vi "Batch-Import-User-Channels Group.vi"(8 "error in (no error)":errorcluster, 11 "Node Ptr":T1 format="%.0x") -> (0 "error out":errorcluster)   [LabVIEW 2015, in "Batch-Import-User-Channels Custom Device.lvlib"]
uses:
  Batch-Import-User-Channels Custom Device.lvlib
  <vilib>/NI Veristand/Custom Device API/Custom Device Item Ref.ctl
  <vilib>/NI Veristand/Custom Device API/Custom Device Channel.ctl
  <vilib>/NI Veristand/Custom Device API/Custom Device Channel Type.ctl
  <vilib>/NI Veristand/Custom Device API/Custom Device API.lvlib
panel:
  in  "Add Channel Folder":bool
  in  "Add Channel":bool
  in  "Header":cluster{"Section Name":string}={"Section Name"="Item Settings"}
  in  "Description":string
  in  "Name":string
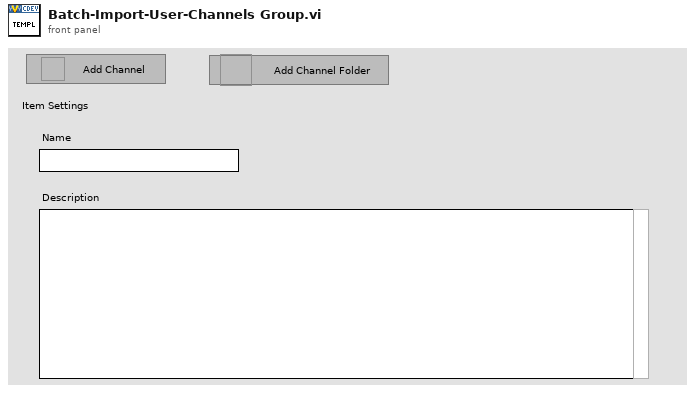
[diagram p1: front panel]
types:
  T1 = typedef "Custom Device API.lvlib/Custom Device Item Ref.ctl" = u64
  T2 = typedef "Custom Device API.lvlib/Custom Device Item Info.ctl" = cluster{"Name":string, "Is Channel":bool, "GUID":string, "Is Waveform":bool}
  T3 = typedef "Custom Device API.lvlib/Custom Device Channel.ctl" = cluster{"Type":T4, "Units":string, "Default Value":dbl, "Faultable":bool, "Scalable":bool}
  T4 = typedef "Custom Device API.lvlib/Custom Device Channel Type.ctl" = enum16{"Input", "Output"}
  T5 = typedef "Custom Device API.lvlib/Custom Device Commands.ctl" = enum16{"Default", "Item renamed", "Shutdown", "Dynamic button pressed"}
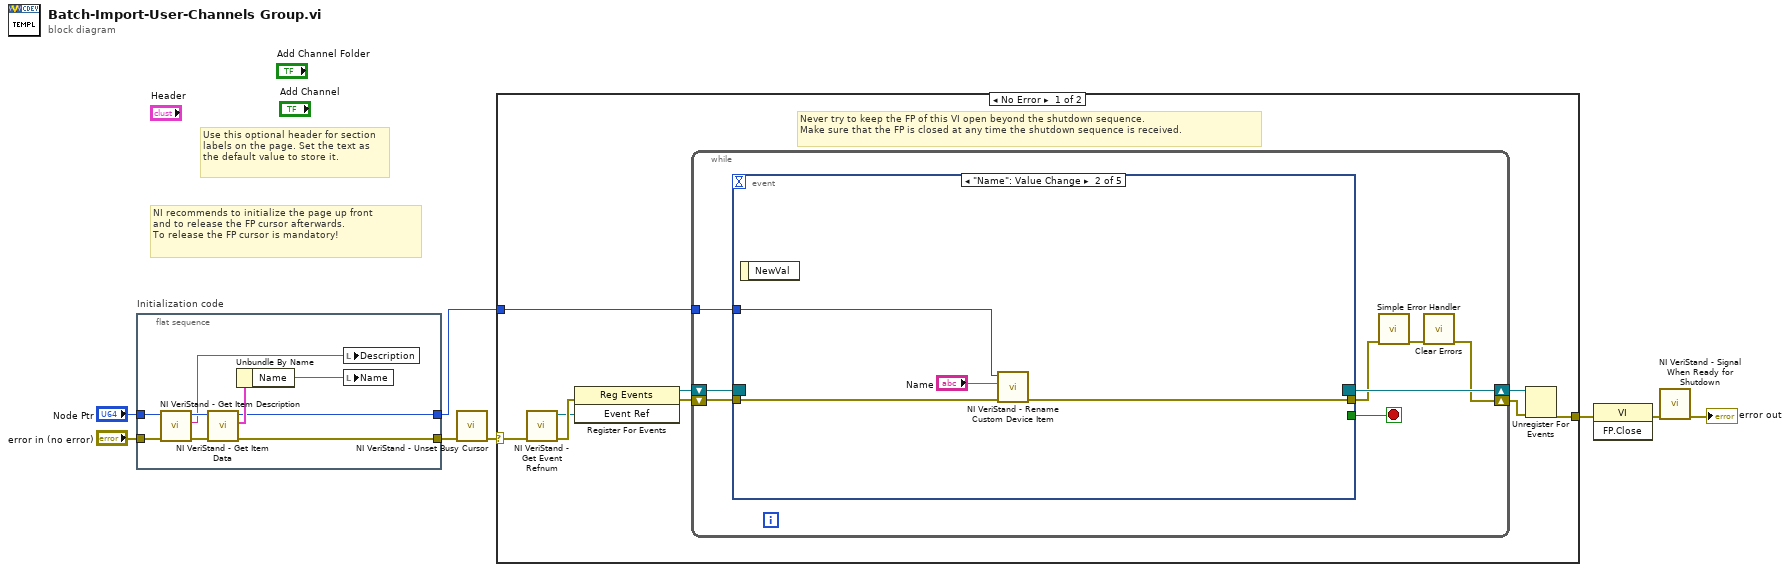
[diagram p0: block diagram]
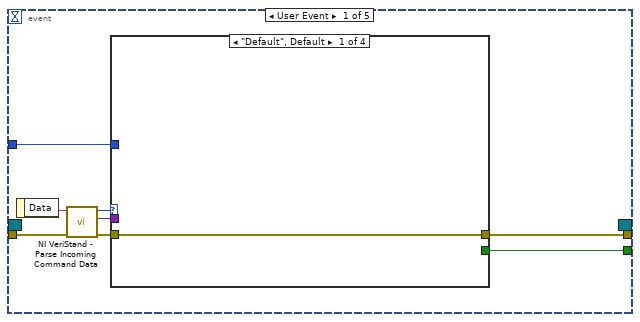
[diagram p2: hidden frame]
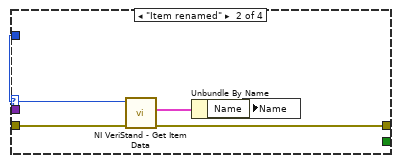
[diagram p3: hidden frame]
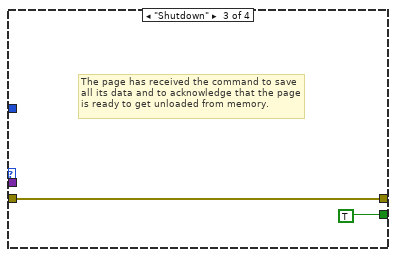
[diagram p4: hidden frame]
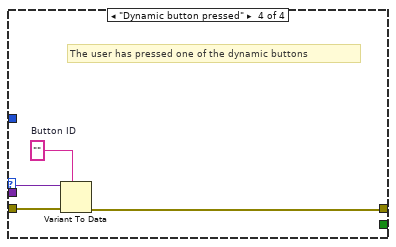
[diagram p5: hidden frame]
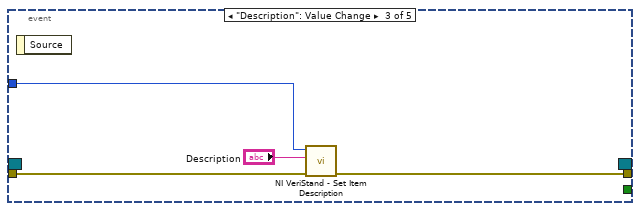
[diagram p6: hidden frame]
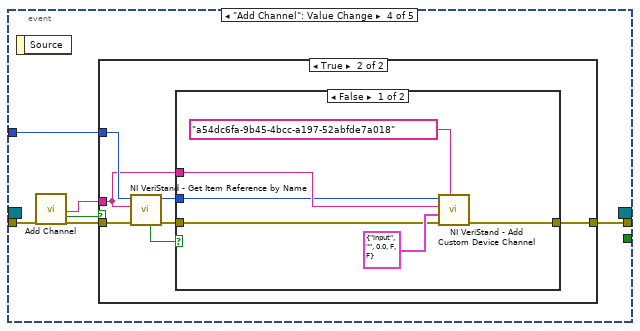
[diagram p7: hidden frame]
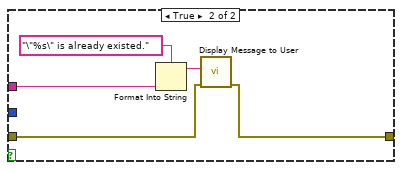
[diagram p9: hidden frame]
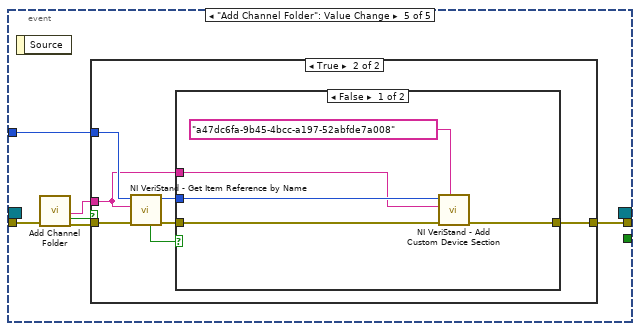
[diagram p10: hidden frame]
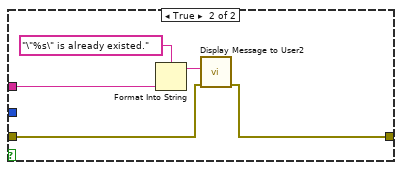
[diagram p12: hidden frame]
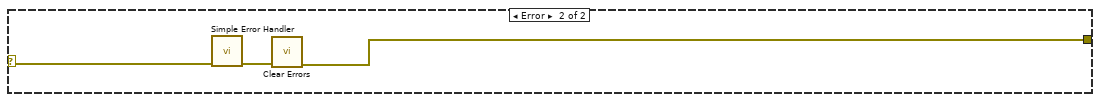
[diagram p13: hidden frame]
diagram:
  # "Use this optional header for section labels on the page. Set the text as the default value to store it."
  # "NI recommends to initialize the page up front\nand to release the FP cursor afterwards.\nTo release the FP cursor is mandatory!"
  n1 = flat-sequence "Initialization code" {
    tunnel: "error in (no error)" -> [w16]
    tunnel: "Node Ptr" -> [w15]
    tunnel: [w9] -> w2
    tunnel: [w10] -> w1
    frame #0 {
      n2 = call <vilib>:"NI VeriStand - Get Item Description.vi"("error in (no error)"=w16, "Item Ref in"=w15) -> ("error out"=w13:errorcluster, "Description"=w14:string, "Item Ref out"=w17:T1)  [unwired: 7 out]
      n3 = call <vilib>:"NI VeriStand - Get Item Data.vi"("error in (no error)"=w13, "Item Ref in"=w17) -> ("error out"=w9:errorcluster, "Item Info"=w12:T2, "Item Ref out"=w10:T1)  [unwired: 7 out]
      n4 = Unbundle By Name(w12) -> ("Name"=w11:string)
      n5 = local write "Description"(w14) -> ()
      n6 = local write "Name"(w11) -> ()
    }
  }
  n7 = call <vilib>:"NI VeriStand - Unset Busy Cursor.vi"("error in (no error)"=w2) -> ("error out"=w4:errorcluster)  [unwired: 10 out]
  n8 = case shown="No Error" w4 {
    selector: w4 -> [w18 w114]
    tunnel: [w23 w112] -> w8
    tunnel: w1 -> [w19 _]
    frame No Error {
      # "Never try to keep the FP of this VI open beyond the shutdown sequence.\nMake sure that the FP is closed at any time the shutdown sequence is received."
      n9 = call <vilib>:"NI VeriStand - Get Event Refnum.vi"("error in (no error)"=w18) -> ("error out"=w26:errorcluster, "Event Ref"=w22:refnum<user-event>)  [unwired: 9 out]
      n10 = register-events(error in=w26, w22) -> (reference out=w20:refnum<event-registration>, error out=w21:errorcluster)  [unwired: 1 in]
      n11 = while {
        tunnel: w19 -> [w30]
        shift-right: [w27] -> w24
        shift-left: w21 -> [w33]
        shift-right: [w34] -> w25
        shift-left: w20 -> [w32]
        stop <- w31 stop-if-true
        n12 = event shown="[1] \"Name\": Value Change" {
          selector: w32 -> [_ _ _ _ _]
          dyn-events: [_ _ _ _ _] -> w34
          timeout: _ -> [_ _ _ _ _]
          tunnel: w33 -> [w42 w58 w61 w63 w91]
          tunnel: [w38 _ _ _ _] -> w31
          tunnel: [w37 w57 w60 w65 w92] -> w29
          tunnel: w30 -> [w36 w56 w62 w64 w93]
          event User Event {
            n13 = event-data() -> ("Data"=w41:string)  [unwired: 1 out]
            n14 = call <vilib>:"NI VeriStand - Parse Incoming Command Data.vi"("error in (no error)"=w42, "Incoming data"=w41) -> ("error out"=w40:errorcluster, "Outgoing data"=w35:variant, "Action"=w39:T5)  [unwired: 7 out]
            n15 = case shown="\"Default\", Default" w39 {
              tunnel: w40 -> [w43 w48 w49 w54]
              tunnel: [_ _ TRUE _] -> w38
              tunnel: [w43 w45 w49 w51] -> w37
              tunnel: w36 -> [_ w47 _ _]
              tunnel: w35 -> [_ _ _ w53]
              frame "Default", Default {
              }
              frame "Item renamed" {
                n16 = call <vilib>:"NI VeriStand - Get Item Data.vi"("error in (no error)"=w48, "Item Ref in"=w47) -> ("error out"=w45:errorcluster, "Item Info"=w46:T2)  [unwired: 8 out]
                n17 = Unbundle By Name(w46) -> ("Name"=w44:string)
                n18 = local write "Name"(w44) -> ()
              }
              frame "Shutdown" {
                # "The page has received the command to save all its data and to acknowledge that the page is ready to get unloaded from memory."
              }
              frame "Dynamic button pressed" {
                w52 = ""  # Button ID
                # "The user has pressed one of the dynamic buttons"
                n19 = Variant To Data(error in=w54, type=w52, Variant=w53) -> (error out=w51:errorcluster)  [unwired: 1 out]
              }
            }
          }
          event "Name": Value Change {
            n20 = event-data() -> ()  [unwired: 2 out]
            n21 = call <vilib>:"NI VeriStand - Rename Custom Device Item.vi"("error in (no error)"=w58, "New Name"="Name", "Item Ref in"=w56) -> ("error out"=w57:errorcluster)  [unwired: 1 in, 7 out]
          }
          event "Description": Value Change {
            n22 = event-data() -> ()  [unwired: 2 out]
            n23 = call <vilib>:"NI VeriStand - Set Item Description.vi"("error in (no error)"=w61, "Description"="Description", "Item Ref in"=w62) -> ("error out"=w60:errorcluster)  [unwired: 8 out]
          }
          event "Add Channel": Value Change {
            n24 = event-data() -> ()  [unwired: 2 out]
            n25 = call "Add Channel"("error in (no error)"=w63) -> ("Channel Name"=w67:string, "OK"=w68:bool, "error out"=w66:errorcluster)  [unwired: 16 in]
            n26 = case shown="True" w68 {
              tunnel: w67 -> [_ w72]
              tunnel: w66 -> [w69 w75]
              tunnel: w64 -> [_ w76]
              tunnel: [w69 w71] -> w65
              frame False {
              }
              frame True {
                n27 = call <vilib>:"NI VeriStand - Get Item Reference by Name.vi"("error in (no error)"=w75, "Item Name"=w72, "Parent Ref in"=w76) -> ("error out"=w73:errorcluster, "Parent Ref out"=w70:T1, "Found"=w74:bool)  [unwired: 5 in, 1 out]
                n28 = case shown="False" w74 {
                  tunnel: w73 -> [w81 w84]
                  tunnel: w72 -> [w80 w85]
                  tunnel: [w78 w83] -> w71
                  tunnel: w70 -> [w77 _]
                  frame False {
                    n29 = call <vilib>:"NI VeriStand - Add Custom Device Channel.vi"("GUID (Default Channel)"="a54dc6fa-9b45-4bcc-a197-52abfde7a018", "error in (no error)"=w81, "Channel"=T3 {"Type"=enum."Input", "Units"="", "Default Value"=0.0, "Faultable"=FALSE, "Scalable"=FALSE}, "Channel Name"=w80, "Parent Ref in"=w77) -> ("error out"=w78:errorcluster)  [unwired: 3 in, 3 out]
                  }
                  frame True {
                    n30 = Format Into String(format string="\"%s\" is already existed.", w85) -> (resulting string=w86:string)  [unwired: 2 in, 1 out]
                    n31 = call "Display Message to User"("error in (no error)"=w84, "Message"=w86) -> ("error out"=w83:errorcluster)  [unwired: 8 in, 1 out]
                  }
                }
              }
            }
          }
          event "Add Channel Folder": Value Change {
            n32 = event-data() -> ()  [unwired: 2 out]
            n33 = call "Add Channel Folder"("error in (no error)"=w91) -> ("Channel Folder Name"=w89:string, "OK"=w88:bool, "error out"=w90:errorcluster)  [unwired: 16 in]
            n34 = case shown="True" w88 {
              tunnel: w89 -> [_ w97]
              tunnel: w90 -> [w94 w100]
              tunnel: w93 -> [_ w101]
              tunnel: [w94 w96] -> w92
              frame False {
              }
              frame True {
                n35 = call <vilib>:"NI VeriStand - Get Item Reference by Name.vi"("error in (no error)"=w100, "Item Name"=w97, "Parent Ref in"=w101) -> ("error out"=w98:errorcluster, "Parent Ref out"=w95:T1, "Found"=w99:bool)  [unwired: 5 in, 1 out]
                n36 = case shown="False" w99 {
                  tunnel: w98 -> [w104 w108]
                  tunnel: w97 -> [w105 w109]
                  tunnel: [w102 w107] -> w96
                  tunnel: w95 -> [w106 _]
                  frame False {
                    n37 = call <vilib>:"NI VeriStand - Add Custom Device Section.vi"("GUID (Default Section)"="a47dc6fa-9b45-4bcc-a197-52abfde7a008", "error in (no error)"=w104, "Section Name"=w105, "Parent Ref in"=w106) -> ("error out"=w102:errorcluster)  [unwired: 4 in, 3 out]
                  }
                  frame True {
                    n38 = Format Into String(format string="\"%s\" is already existed.", w109) -> (resulting string=w110:string)  [unwired: 2 in, 1 out]
                    n39 = call "Display Message to User2"("error in (no error)"=w108, "Message"=w110) -> ("error out"=w107:errorcluster)  [unwired: 8 in, 1 out]
                  }
                }
              }
            }
          }
        }
        n40 = call <vilib>:"Simple Error Handler.vi"("error in (no error)"=w29) -> ("error out"=w28:errorcluster)  [unwired: 1 in, 7 out]
        n41 = call <vilib>:"Clear Errors.vi"("error in (no error)"=w28) -> ("error out"=w27:errorcluster)  [unwired: 1 in, 5 out]
      }
      n42 = Unregister For Events(event registration refnum=w25, error in=w24) -> (error out=w23:errorcluster)
    }
    frame Error {
      n43 = call <vilib>:"Simple Error Handler.vi"("error in (no error)"=w114) -> ("error out"=w113:errorcluster)  [unwired: 1 in, 7 out]
      n44 = call <vilib>:"Clear Errors.vi"("error in (no error)"=w113) -> ("error out"=w112:errorcluster)  [unwired: 1 in, 5 out]
    }
  }
  n45 = invoke class="VI" method="FP.Close"(error in=w8) -> (error out=w7:errorcluster)  [unwired: 2 in, 2 out]
  n46 = call <vilib>:"NI VeriStand - Signal When Ready for Shutdown.vi"("error in (no error)"=w7) -> ("error out"=→"error out":errorcluster)  [unwired: 10 out]
